vi "daxpy.vi"(4 "incy":i32, 6 "incx":i32, 7 "n":i32, 8 "da":dbl, 10 "dy":dbl[](array[numeric]), 11 "dx":dbl[](array[numeric])) -> (3 "daxpy_result":dbl[](array[numeric]))   [LabVIEW 2014]
panel:
  out "mp1":i32
  out "m":i32=1
  out "ix":i32=1
  out "iy":i32=1
  out "daxpy result":dbl[](array[numeric])
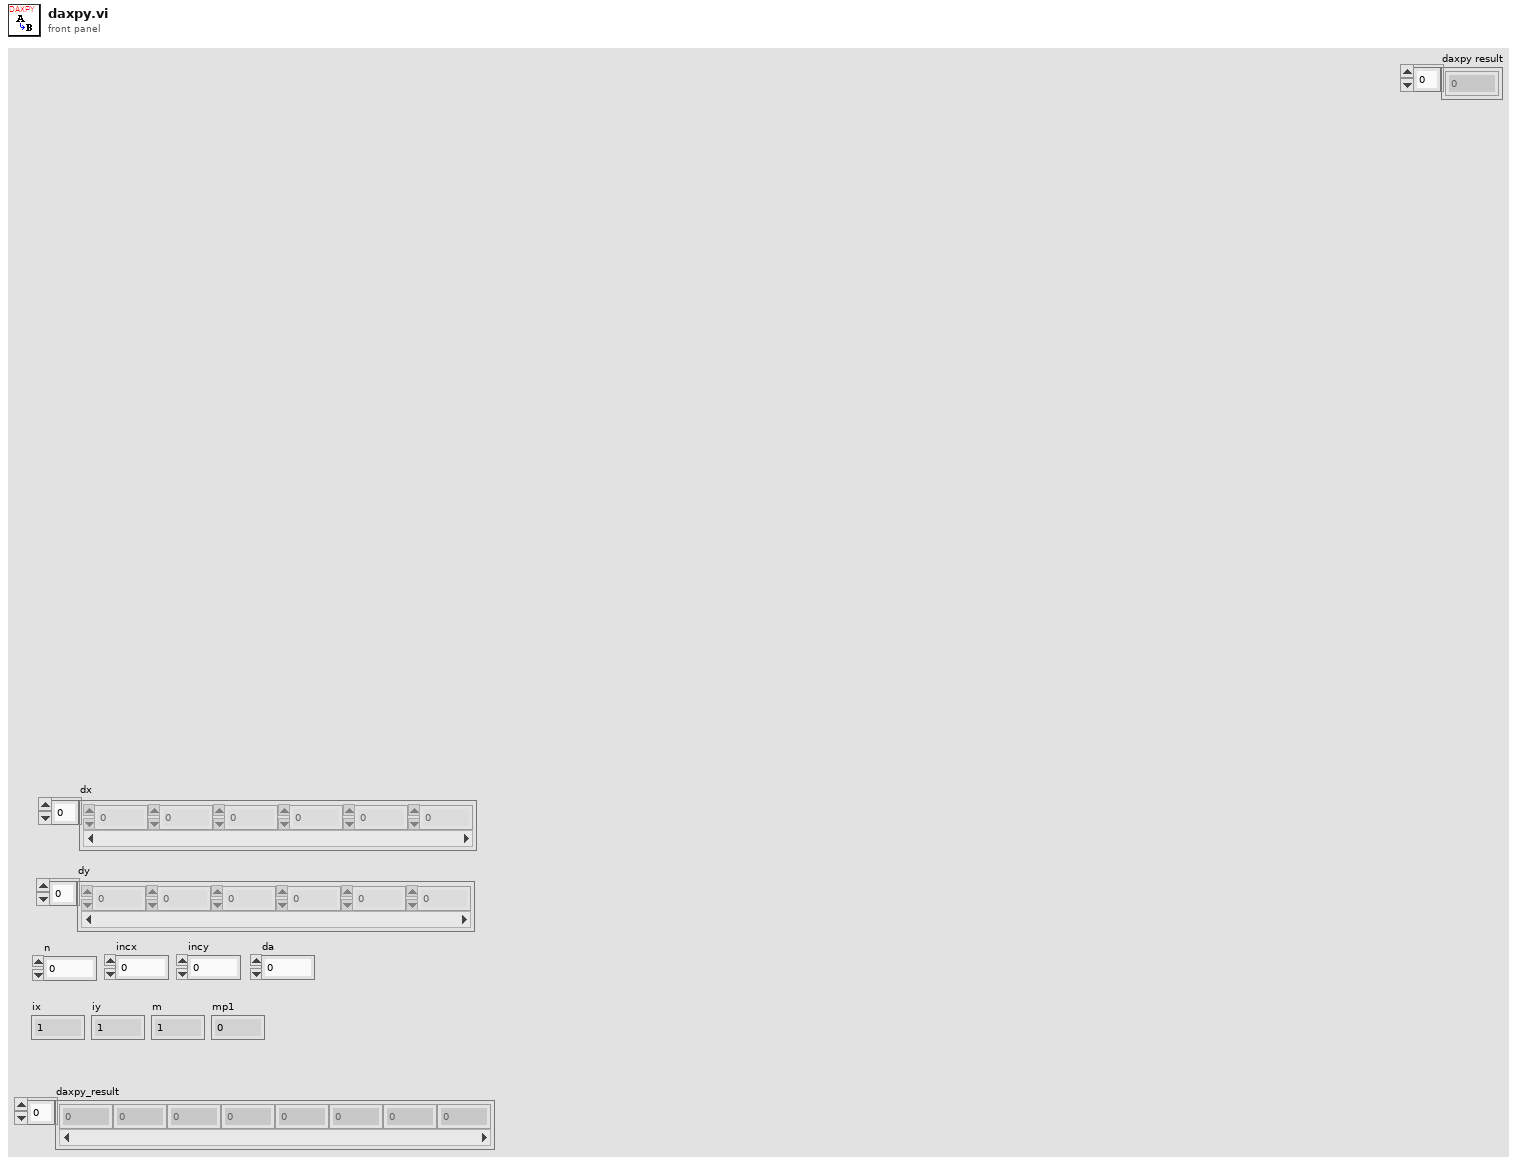
[diagram p1: front panel]
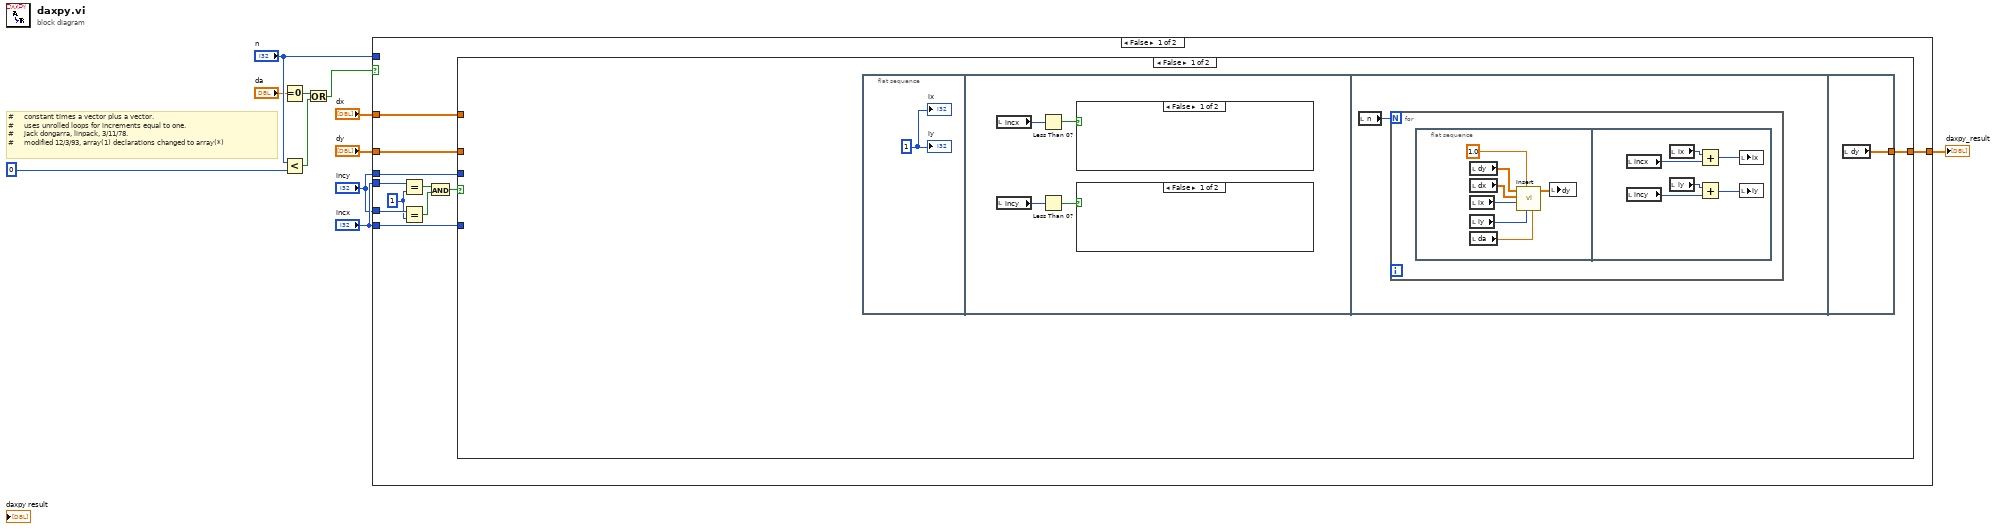
[diagram p0: block diagram]
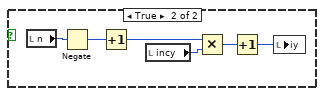
[diagram p2: hidden frame]
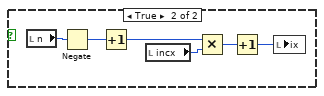
[diagram p3: hidden frame]
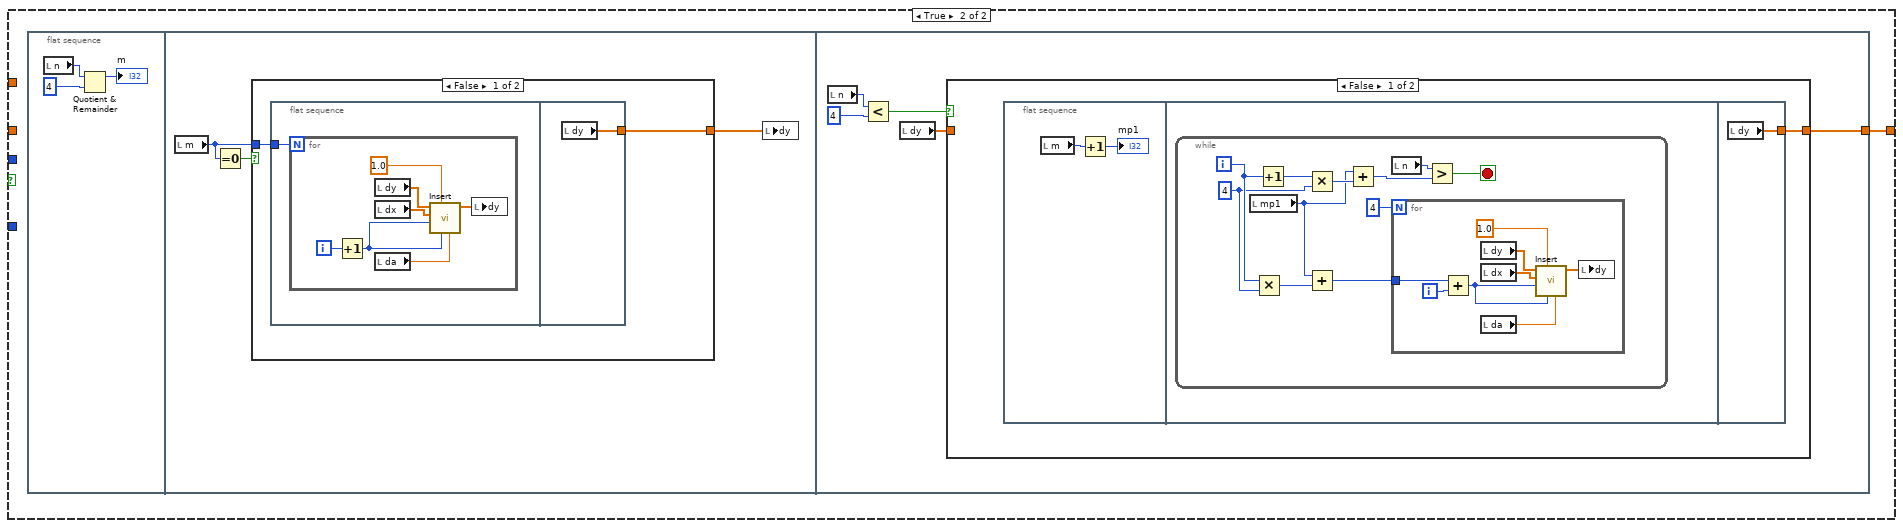
[diagram p4: hidden frame]
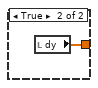
[diagram p5: hidden frame]
diagram:
  # "#     constant times a vector plus a vector.\n#     uses unrolled loops for increments equal to one.\n#     jack dongarra, linpack, 3/11/78.\n#     modified 12/3/93, array(1) declarations changed to array(*)"
  n1 = Equal To 0?(x="da") -> (x = 0?=w1:bool)
  n2 = Less?(x="n", y=0) -> (x < y?=w11:bool)
  n3 = Or(x=w1, y=w11) -> (x .or. y?=w2:bool)
  n4 = case shown="False" w2 {
    tunnel: "dy" -> [w17 w104]
    tunnel: [w12 w104] -> w4
    tunnel: "incx" -> [w22 _]
    tunnel: "dx" -> [w18 _]
    tunnel: "incy" -> [w21 _]
    tunnel: "n" -> [_ _]
    tunnel: "incx" -> [w20 _]
    tunnel: "incy" -> [w19 _]
    frame False {
      w16 = 1
      n5 = Equal?(x=w22, y=w16) -> (x = y?=w15:bool)
      n6 = Equal?(x=w21, y=w16) -> (x = y?=w14:bool)
      n7 = And(x=w15, y=w14) -> (x .and. y?=w13:bool)
      n8 = case shown="False" w13 {
        tunnel: w20 -> [_ _]
        tunnel: w19 -> [_ _]
        tunnel: w18 -> [_ _]
        tunnel: w17 -> [_ _]
        tunnel: [w23 w56] -> w12
        frame False {
          n9 = flat-sequence {
            tunnel: [w55] -> w23
            frame #0 {
              w24 = 1
              "ix" <- w24
              "iy" <- w24
            }
            frame #1 {
              n10 = local read "incx"() -> (w28:i32)
              n11 = local read "incy"() -> (w25:i32)
              n12 = Less Than 0?(x=w28) -> (x < 0?=w27:bool)
              n13 = Less Than 0?(x=w25) -> (x < 0?=w26:bool)
              n14 = case shown="False" w27 {
                frame False {
                }
                frame True {
                  n15 = local read "n"() -> (w40:i32)
                  n16 = Negate(x=w40) -> (-x=w39:i32)
                  n17 = Increment(x=w39) -> (x+1=w38:i32)
                  n18 = local read "incx"() -> (w37:i32)
                  n19 = Multiply(x=w38, y=w37) -> (x*y=w36:i32)
                  n20 = Increment(x=w36) -> (x+1=w35:i32)
                  n21 = local write "ix"(w35) -> ()
                }
              }
              n22 = case shown="False" w26 {
                frame False {
                }
                frame True {
                  n23 = local read "n"() -> (w34:i32)
                  n24 = Negate(x=w34) -> (-x=w33:i32)
                  n25 = Increment(x=w33) -> (x+1=w32:i32)
                  n26 = local read "incy"() -> (w31:i32)
                  n27 = Multiply(x=w32, y=w31) -> (x*y=w30:i32)
                  n28 = Increment(x=w30) -> (x+1=w29:i32)
                  n29 = local write "iy"(w29) -> ()
                }
              }
            }
            frame #2 {
              n30 = local read "n"() -> (w41:i32)
              n31 = for {
                N: w41 -> [_]
                n32 = flat-sequence {
                  frame #0 {
                    n33 = local read "dy"() -> (w46:dbl[])
                    n34 = local read "dx"() -> (w45:dbl[])
                    n35 = local read "ix"() -> (w48:i32)
                    n36 = local read "iy"() -> (w47:i32)
                    n37 = local read "da"() -> (w42:dbl)
                    n38 = call "Insert.vi"("da"=w42, "iy"=w47, "dy weight"=1.0, "ix"=w48, "dx"=w45, "dy in"=w46) -> ("dy out"=w44:dbl[])  [unwired: 5 in]
                    n39 = local write "dy"(w44) -> ()
                  }
                  frame #1 {
                    n40 = local read "incx"() -> (w53:i32)
                    n41 = local read "incy"() -> (w50:i32)
                    n42 = local read "ix"() -> (w54:i32)
                    n43 = local read "iy"() -> (w49:i32)
                    n44 = Add(x=w54, y=w53) -> (x+y=w52:i32)
                    n45 = Add(x=w49, y=w50) -> (x+y=w51:i32)
                    n46 = local write "ix"(w52) -> ()
                    n47 = local write "iy"(w51) -> ()
                  }
                }
              }
            }
            frame #3 {
              n48 = local read "dy"() -> (w55:dbl[])
            }
          }
        }
        frame True {
          n49 = flat-sequence {
            tunnel: [w75] -> w56
            frame #0 {
              n50 = local read "n"() -> (w58:i32)
              n51 = Quotient & Remainder(x=w58, y=4) -> (x-y*floor(x/y)=→"m":i32)  [unwired: 1 out]
            }
            frame #1 {
              n52 = local read "m"() -> (w61:i32)
              n53 = Equal To 0?(x=w61) -> (x = 0?=w62:bool)
              n54 = case shown="False" w62 {
                tunnel: [w63 w74] -> w60
                tunnel: w61 -> [w64 _]
                frame False {
                  n55 = flat-sequence {
                    tunnel: w64 -> [w65]
                    tunnel: [w73] -> w63
                    frame #0 {
                      n56 = for {
                        N: w65 -> [_]
                        i -> [w72]
                        n57 = Increment(x=w72) -> (x+1=w71:i32)
                        n58 = local read "dy"() -> (w69:dbl[])
                        n59 = local read "dx"() -> (w70:dbl[])
                        n60 = local read "da"() -> (w66:dbl)
                        n61 = call "Insert.vi"("da"=w66, "iy"=w71, "dy weight"=1.0, "ix"=w71, "dx"=w70, "dy in"=w69) -> ("dy out"=w68:dbl[])  [unwired: 5 in]
                        n62 = local write "dy"(w68) -> ()
                      }
                    }
                    frame #1 {
                      n63 = local read "dy"() -> (w73:dbl[])
                    }
                  }
                }
                frame True {
                  n64 = local read "dy"() -> (w74:dbl[])
                }
              }
              n65 = local write "dy"(w60) -> ()
            }
            frame #2 {
              n66 = local read "n"() -> (w78:i32)
              n67 = Less?(x=w78, y=4) -> (x < y?=w77:bool)
              n68 = local read "dy"() -> (w79:dbl[])
              n69 = case shown="False" w77 {
                tunnel: w79 -> [_ w103]
                tunnel: [w80 w103] -> w75
                frame False {
                  n70 = flat-sequence {
                    tunnel: [w102] -> w80
                    frame #0 {
                      n71 = local read "m"() -> (w82:i32)
                      n72 = Increment(x=w82) -> (x+1=→"mp1":i32)
                    }
                    frame #1 {
                      n73 = while {
                        i -> [w86]
                        stop <- w89 stop-if-true
                        w85 = 4
                        n74 = local read "mp1"() -> (w84:i32)
                        n75 = Multiply(x=w86, y=w85) -> (x*y=w87:i32)
                        n76 = Increment(x=w86) -> (x+1=w93:i32)
                        n77 = Multiply(x=w93, y=w85) -> (x*y=w92:i32)
                        n78 = Add(x=w84, y=w87) -> (x+y=w83:i32)
                        n79 = Add(x=w84, y=w92) -> (x+y=w91:i32)
                        n80 = local read "n"() -> (w90:i32)
                        n81 = for {
                          N: 4 -> [_]
                          tunnel: w83 -> [w101]
                          i -> [w100]
                          n82 = Add(x=w101, y=w100) -> (x+y=w99:i32)
                          n83 = local read "dy"() -> (w97:dbl[])
                          n84 = local read "dx"() -> (w96:dbl[])
                          n85 = local read "da"() -> (w94:dbl)
                          n86 = call "Insert.vi"("da"=w94, "iy"=w99, "dy weight"=1.0, "ix"=w99, "dx"=w96, "dy in"=w97) -> ("dy out"=w98:dbl[])  [unwired: 5 in]
                          n87 = local write "dy"(w98) -> ()
                        }
                        n88 = Greater?(x=w90, y=w91) -> (0:w89:bool)
                      }
                    }
                    frame #2 {
                      n89 = local read "dy"() -> (w102:dbl[])
                    }
                  }
                }
                frame True {
                }
              }
            }
          }
        }
      }
    }
    frame True {
    }
  }
  "daxpy_result" <- w4
